vi "CTB6.vi"() -> ()   [LabVIEW 2015]
uses:
  <vilib>/Instr/_visa.llb/VISA Configure Serial Port (Instr).vi
  <vilib>/Utility/file.llb/Write Delimited Spreadsheet (I64).vi
panel:
  out "CH8":i32[](graph)
  out "CH7":i32[](graph)
  out "CH6":i32[](graph)
  out "CH5":i32[](graph)
  out "CH4":i32[](graph)
  out "CH3":i32[](graph)
  out "CH2":i32[](graph)
  out "CH1":i32[](graph)
  in  "tiempo de muestreo":u32
  in  "timeout (10sec)":u32=10000
  in  "baud rate (9600)":u32=9600
  in  "VISA resource name 2":refnum<visa-resource-name>
  in  "Archivo":path
  out "Muestras":i32
  in  "?":bool
  out "read buffer":string
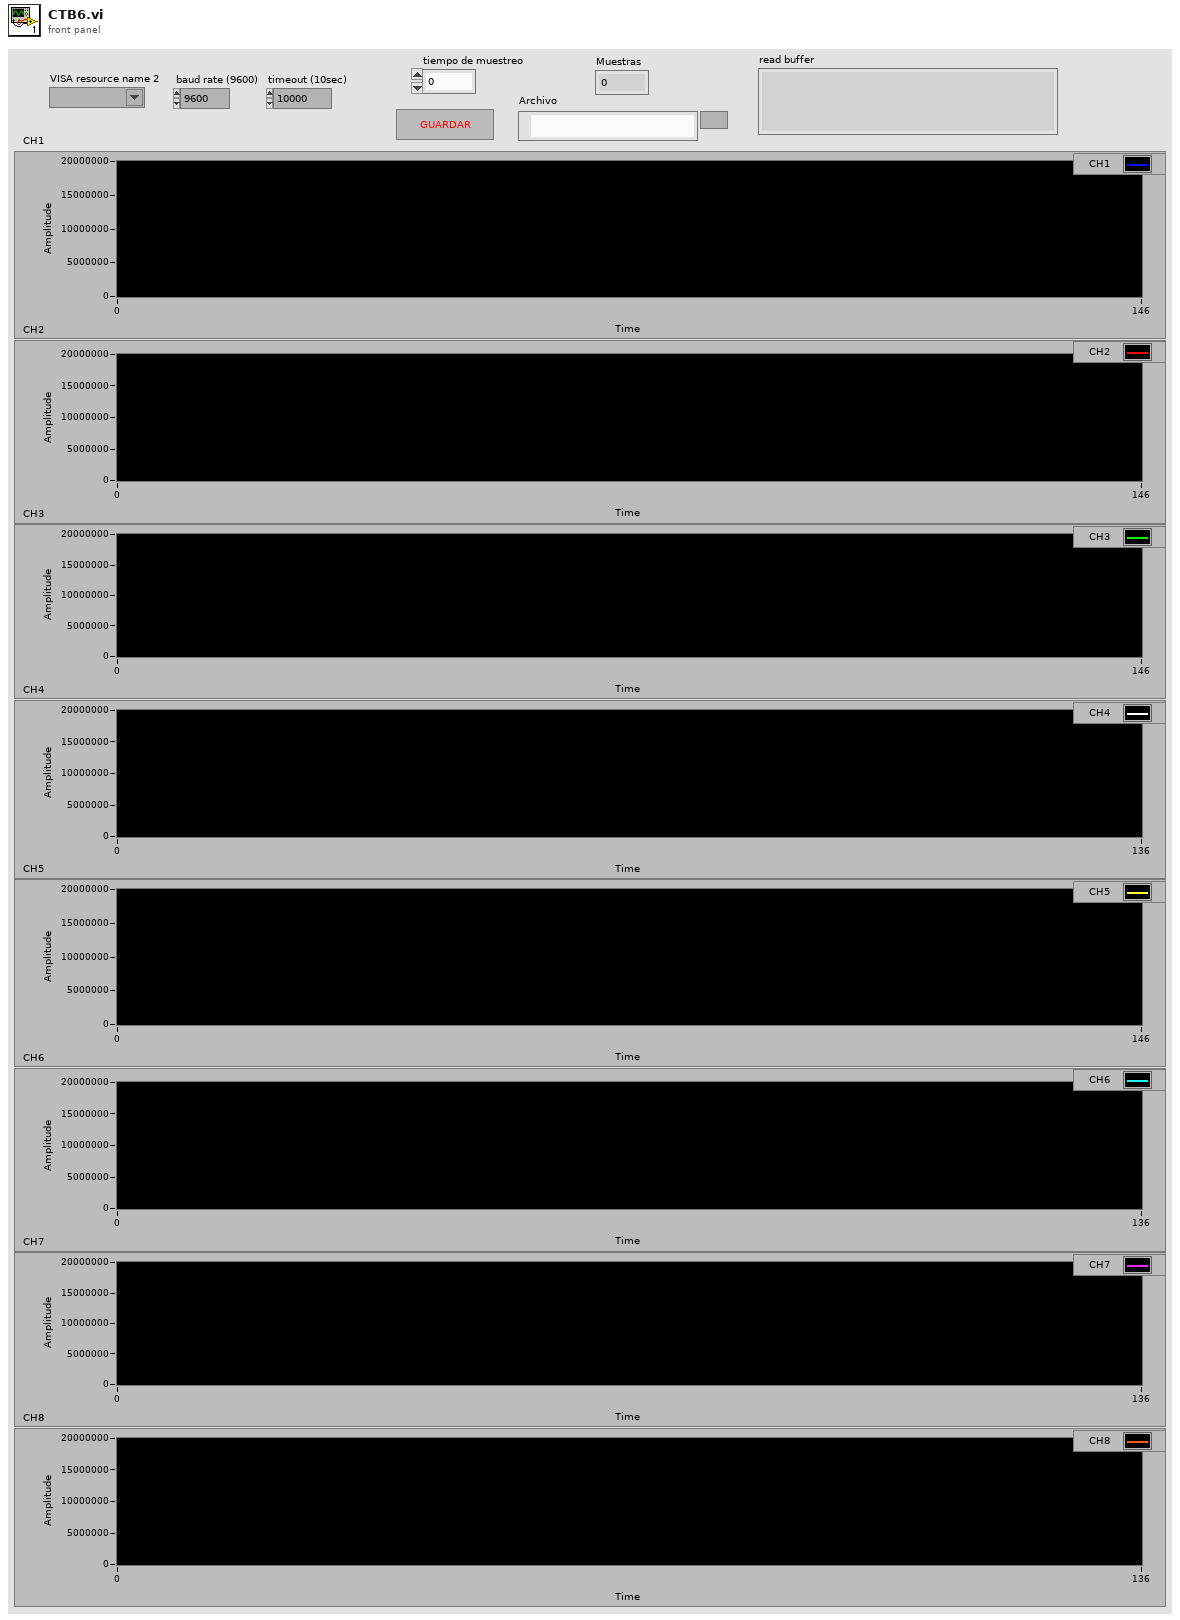
[diagram p1: front panel]
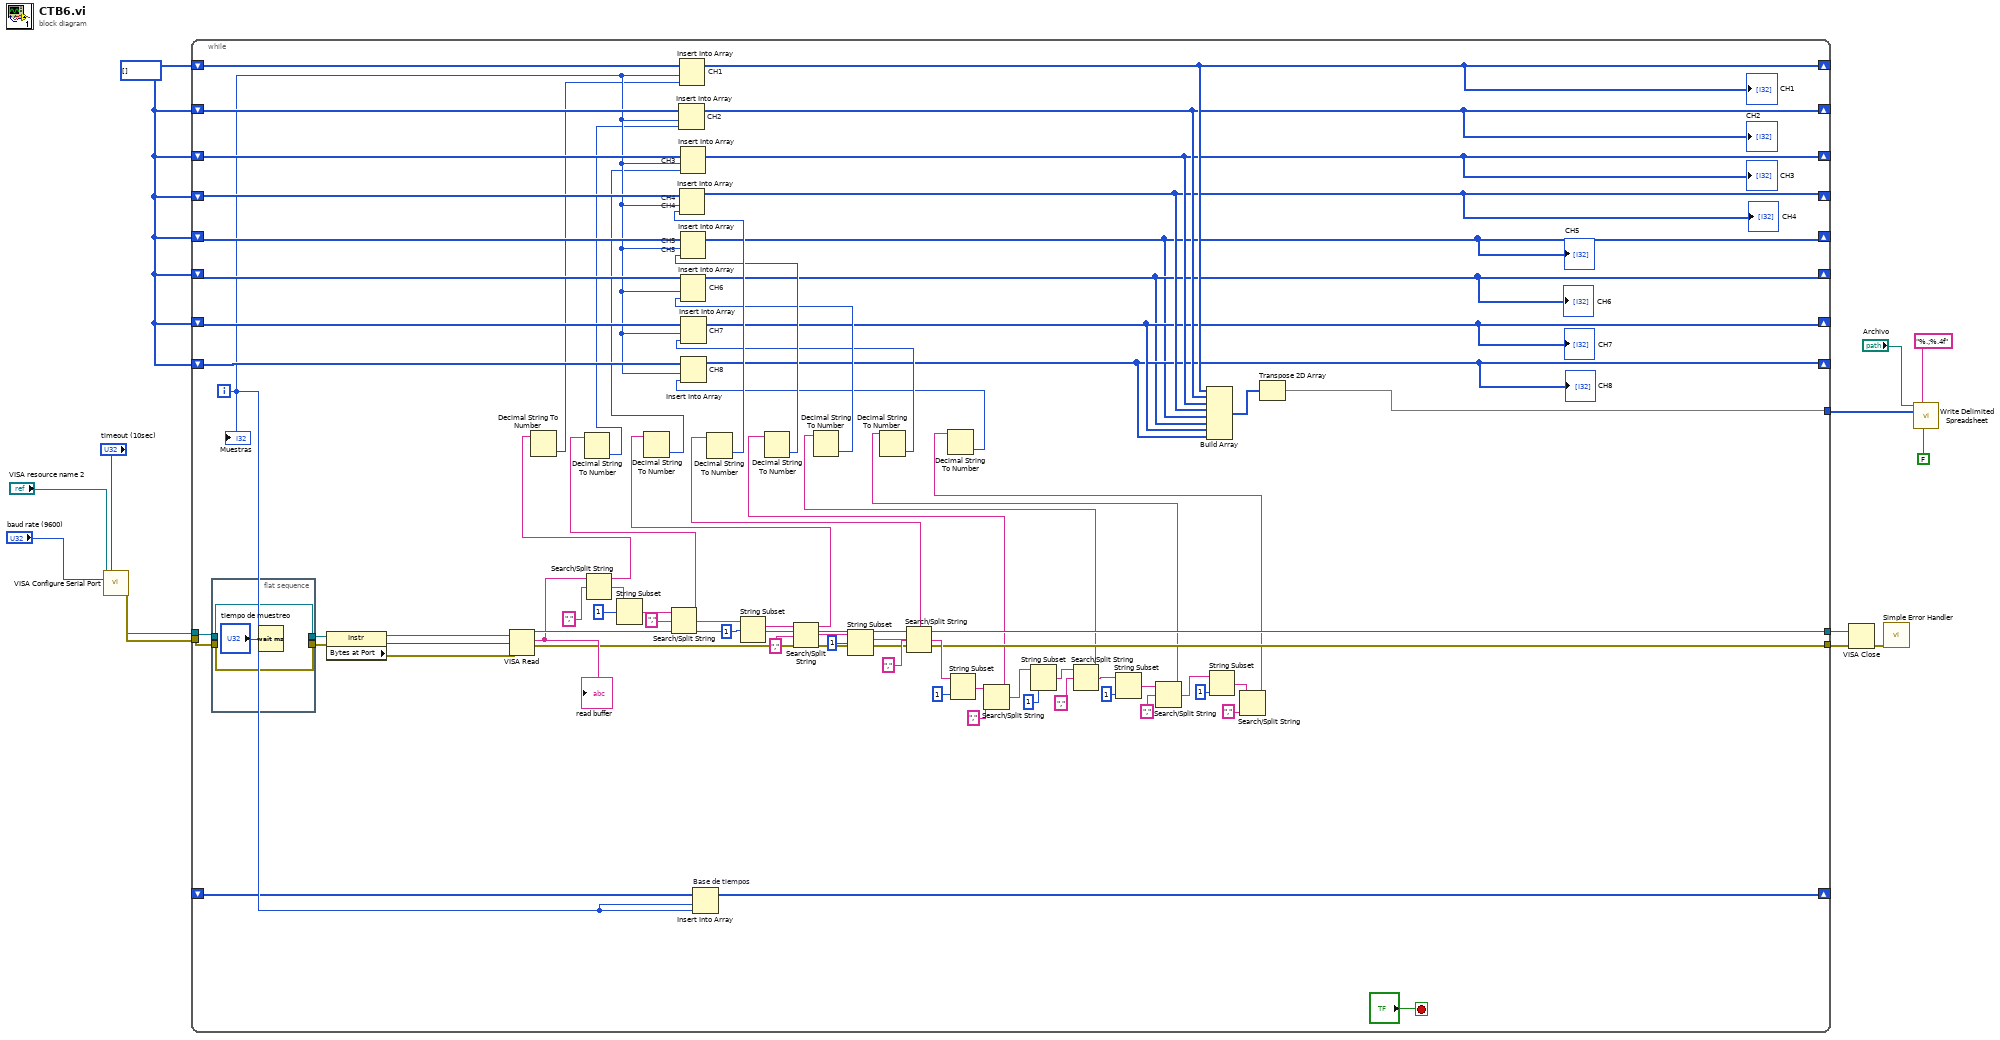
[diagram p0: block diagram]
diagram:
  w2 = i32[] []
  n1 = call-poly "VISA Configure Serial Port"("VISA resource name"="VISA resource name 2", "timeout (10sec)"="timeout (10sec)", "baud rate (9600)"="baud rate (9600)") -> ("VISA resource name out"=w5:refnum<visa-resource-name>, "error out"=w6:errorcluster)  [unwired: 11 in]
  n2 = while {
    shift-right: [w21] -> _
    shift-left: w2 -> [w45]
    shift-right: [w20] -> _
    shift-left: w2 -> [w84]
    shift-right: [w19] -> _
    shift-left: w2 -> [w82]
    shift-right: [w18] -> _
    shift-left: w2 -> [w77]
    shift-right: [w14] -> _
    shift-left: w2 -> [w76]
    shift-right: [w15] -> _
    shift-left: w2 -> [w70]
    shift-right: [w17] -> _
    shift-left: w2 -> [w69]
    shift-right: [w16] -> _
    shift-left: w2 -> [w68]
    tunnel: [w46] -> w11
    tunnel: w5 -> [w65]
    tunnel: w6 -> [w64]
    tunnel: [w67] -> w4
    shift-right: [w41] -> _
    shift-left: _ -> [w42]
    tunnel: [w39] -> w1
    i -> [w43]
    stop <- "?" stop-if-true
    n3 = flat-sequence {
      tunnel: w65 -> [w93]
      tunnel: [w93] -> w66
      tunnel: w64 -> [w92]
      tunnel: [w92] -> w63
      frame #0 {
        n4 = Wait (ms)(milliseconds to wait="tiempo de muestreo") -> ()  [unwired: 1 out]
      }
    }
    n5 = property class="Instr"(reference=w66, error in=w63) -> (reference out=w90:refnum<visa-resource-name>, error out=w40:errorcluster, "Bytes at Port"=w89:u32)
    n6 = VISA Read(VISA resource name=w90, byte count=w89, error in (no error)=w40) -> (VISA resource name out=w67:refnum<visa-resource-name>, read buffer=w44:string, error out=w39:errorcluster)  [unwired: 1 out]
    "read buffer" <- w44
    n7 = Search/Split String(string=w44, search string/char (-)=",") -> (substring before match=w37:string, match + rest of string=w86:string)  [unwired: 1 in, 1 out]
    n8 = Decimal String To Number(string=w37) -> (number=w36:i32)  [unwired: 2 in, 1 out]
    n9 = String Subset(string=w86, offset (0)=1) -> (substring=w81:string)  [unwired: 1 in]
    n10 = Search/Split String(string=w81, search string/char (-)=",") -> (substring before match=w35:string, match + rest of string=w79:string)  [unwired: 1 in, 1 out]
    n11 = Decimal String To Number(string=w35) -> (number=w34:i32)  [unwired: 2 in, 1 out]
    n12 = Insert Into Array "CH2"(array=w84, index=w43, new element=w34) -> (w20:i32[])
    "CH2" <- w20
    n13 = Insert Into Array "CH1"(array=w45, index=w43, new element=w36) -> (w21:i32[])
    "CH1" <- w21
    n14 = Insert Into Array "Base de tiempos"(array=w42, index=w43, new element=w43) -> (w41:i32[])
    n15 = String Subset(string=w79, offset (0)=1) -> (substring=w62:string)  [unwired: 1 in]
    n16 = Search/Split String(string=w62, search string/char (-)=",") -> (substring before match=w33:string, match + rest of string=w74:string)  [unwired: 1 in, 1 out]
    n17 = Decimal String To Number(string=w33) -> (number=w32:i32)  [unwired: 2 in, 1 out]
    n18 = Insert Into Array "CH3"(array=w82, index=w43, new element=w32) -> (w19:i32[])
    "CH3" <- w19
    n19 = String Subset(string=w74, offset (0)=1) -> (substring=w61:string)  [unwired: 1 in]
    n20 = Search/Split String(string=w61, search string/char (-)=",") -> (substring before match=w31:string, match + rest of string=w71:string)  [unwired: 1 in, 1 out]
    n21 = Decimal String To Number(string=w31) -> (number=w30:i32)  [unwired: 2 in, 1 out]
    n22 = Insert Into Array "CH4\nCH4"(array=w77, index=w43, new element=w30) -> (w18:i32[])
    "CH4" <- w18
    n23 = String Subset(string=w71, offset (0)=1) -> (substring=w59:string)  [unwired: 1 in]
    n24 = Search/Split String(string=w59, search string/char (-)=",") -> (substring before match=w29:string, match + rest of string=w55:string)  [unwired: 1 in, 1 out]
    n25 = Decimal String To Number(string=w29) -> (number=w28:i32)  [unwired: 2 in, 1 out]
    n26 = Insert Into Array "CH5\nCH5"(array=w76, index=w43, new element=w28) -> (w14:i32[])
    "CH5" <- w14
    n27 = String Subset(string=w55, offset (0)=1) -> (substring=w56:string)  [unwired: 1 in]
    n28 = Search/Split String(string=w56, search string/char (-)=",") -> (substring before match=w27:string, match + rest of string=w51:string)  [unwired: 1 in, 1 out]
    n29 = Decimal String To Number(string=w27) -> (number=w26:i32)  [unwired: 2 in, 1 out]
    n30 = Insert Into Array "CH6"(array=w70, index=w43, new element=w26) -> (w15:i32[])
    "CH6" <- w15
    n31 = String Subset(string=w51, offset (0)=1) -> (substring=w52:string)  [unwired: 1 in]
    n32 = Search/Split String(string=w52, search string/char (-)=",") -> (substring before match=w25:string, match + rest of string=w47:string)  [unwired: 1 in, 1 out]
    n33 = Decimal String To Number(string=w25) -> (number=w24:i32)  [unwired: 2 in, 1 out]
    n34 = Insert Into Array "CH7"(array=w69, index=w43, new element=w24) -> (w17:i32[])
    "CH7" <- w17
    n35 = String Subset(string=w47, offset (0)=1) -> (substring=w48:string)  [unwired: 1 in]
    n36 = Search/Split String(string=w48, search string/char (-)=",") -> (substring before match=w23:string)  [unwired: 1 in, 2 out]
    n37 = Decimal String To Number(string=w23) -> (number=w22:i32)  [unwired: 2 in, 1 out]
    n38 = Insert Into Array "CH8"(array=w68, index=w43, new element=w22) -> (w16:i32[])
    "CH8" <- w16
    n39 = Build Array "Build Array"(w21, w20, w19, w18, w14, w15, w17, w16) -> (w38:i32[][])
    n40 = Transpose 2D Array(2D array=w38) -> (transposed array=w46:i32[][])
    "Muestras" <- w43
  }
  n41 = VISA Close(VISA resource name=w4, error in (no error)=w1) -> (error out=w3:errorcluster)
  n42 = call <vilib>:"Simple Error Handler.vi"("error in (no error)"=w3) -> ()  [unwired: 4 in, 5 out]
  n43 = call-poly <vilib>:"Write Delimited Spreadsheet.vi"("file path (dialog if empty)"="Archivo", "format (%d)"="%.;%.4f" ("format (%.3f)"), "2D data"=w11, "transpose? (F)"=FALSE ("transpose? (no:F)")) -> ()  [unwired: 10 in, 2 out]
